vi "5209_Set_Frequency.vi"(2 "error in (no error)":errorcluster, 3 "Frequency":dbl, 4 "VISA resource name":refnum<visa-resource-name>) -> (0 "error out":errorcluster, 1 "VISA resource name out":refnum<visa-resource-name>)   [LabVIEW 2015]
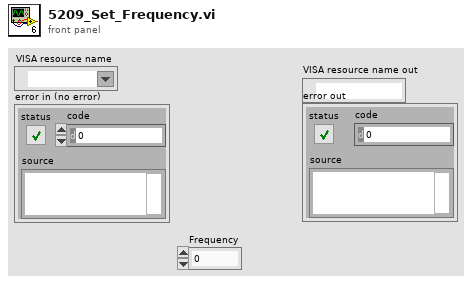
[diagram p1: front panel]
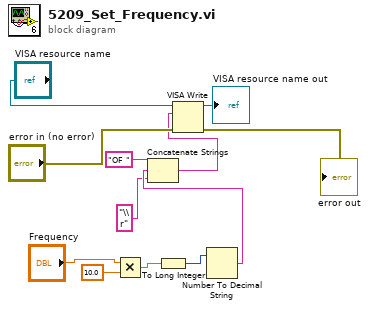
[diagram p0: block diagram]
diagram:
  n1 = Multiply(x="Frequency", y=10.0) -> (x*y=w5:dbl)
  n2 = To Long Integer(number=w5) -> (32bit integer=w4:i32)
  n3 = Number To Decimal String(number=w4) -> (decimal integer string=w2:string)  [unwired: 1 in]
  n4 = Concatenate Strings("OF " ("string"), w2, "\\r" ("string")) -> (w3:string)
  n5 = VISA Write(VISA resource name="VISA resource name", write buffer=w3, error in (no error)="error in (no error)") -> (VISA resource name out=→"VISA resource name out":refnum<visa-resource-name>, error out=→"error out":errorcluster)  [unwired: 1 out]
